vi "Photobleach Custom.vi"(8 "error in (no error)":errorcluster, 9 "Shutter Enable":bool[](array[boolean]), 10 "Length (mm)":dbl, 11 "Application in":refnum<class "Application.lvclass">) -> (0 "error out":errorcluster, 3 "Application out":refnum<class "Application.lvclass">)   [LabVIEW 2018, in "Application.lvlib" / "Application.lvclass"]
uses:
  Application.lvclass
  Application Messages/Close Shutter Msg/Close Shutter Msg.lvclass
  C:/Program Files/National Instruments/LabVIEW 2018/vi.lib/ActorFramework/Message/Message.lvclass
  Application.lvclass/Application.ctl
  Hardware/Laser Messages/Set Laser Power Msg/Set Laser Power Msg.lvclass/Set Laser Power Msg.ctl
  <vilib>/ActorFramework/Message Enqueuer/Message Enqueuer.lvclass/Message Enqueuer.ctl
  Hardware/Stage Controller Messages/Photobleach Custom Msg/Photobleach Custom Msg.lvclass/Photobleach Custom Msg.ctl
  <vilib>/ActorFramework/Message Enqueuer/Enqueue.vi
  Hardware/Laser Messages/Set Laser Power Msg/Set Laser Power Msg.lvclass
  Hardware/Stage Controller Messages/Photobleach Custom Msg/Photobleach Custom Msg.lvclass
  Resources/GLOBAL/GLOBAL Time-critical.vi
  <vilib>/ActorFramework/Message Priority Queue/Priority Enqueue.vi
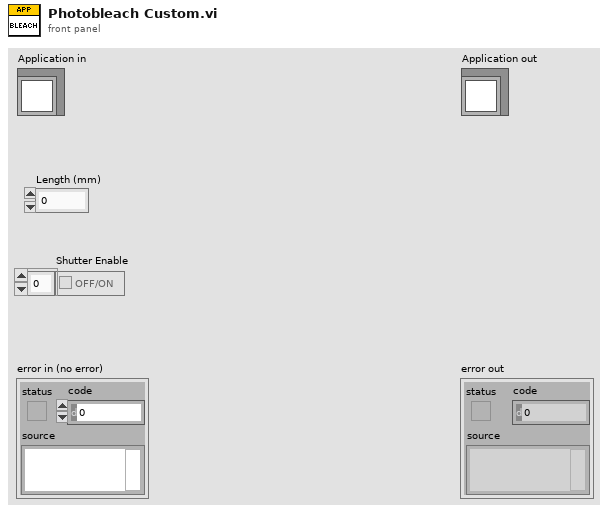
[diagram p1: front panel]
types:
  T1 = typedef "Shutter Configuration.ctl" = cluster{"IO Line":tag, "Name":string, "Wavelength":u16, "Max rate (Hz)":dbl}
  T2 = typedef "Laser Configuration.ctl" = cluster{"Serial Port":refnum<visa-resource-name>, "Laser Type":enum16{"Disable", "Laser Quantum", "Coherent OBIS", "PRM1-Z8", "Coherent HOPS"}, "Polarizer Amplitude":dbl, "Polarizer Theta Zero":dbl, "Wavelength":u16}
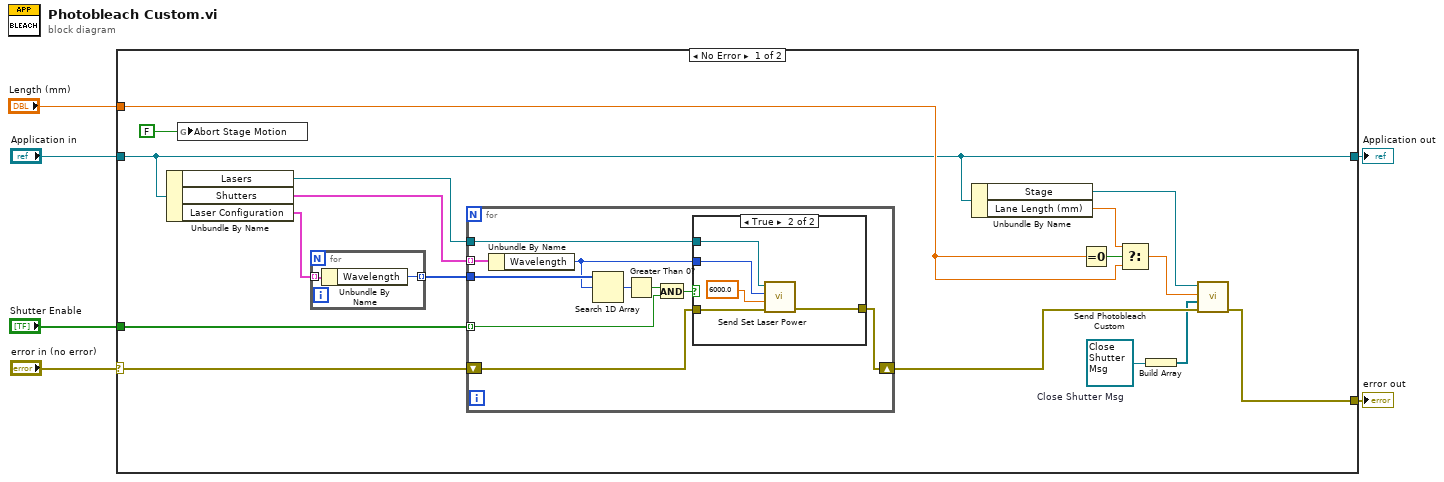
[diagram p0: block diagram]
diagram:
  n1 = case shown="No Error" "error in (no error)" {
    selector: "error in (no error)" -> [w16 w43]
    tunnel: [w22 w43] -> w5
    tunnel: [w14 w42] -> w3
    tunnel: "Application in" -> [w14 w42]
    tunnel: "Length (mm)" -> [w18 _]
    tunnel: "Shutter Enable" -> [w11 _]
    frame No Error {
      w7 = refnum<class "Close Shutter Msg.lvclass"> refnum  # Close Shutter Msg
      n2 = Unbundle By Name(w14) -> ("Lasers"=w13:refnum<class "Message Enqueuer.lvclass">, "Shutters"=w12:T1[], "Laser Configuration"=w10:T2[])
      n3 = global write "GLOBAL Time-critical.vi" "Abort Stage Motion"(FALSE ("Abort Stage Motion")) -> ()
      n4 = for {
        tunnel: w10 -> [w25] mode=indexing
        tunnel: [w24] -> w9 mode=indexing
        n5 = Unbundle By Name(w25) -> ("Wavelength"=w24:u16)
      }
      n6 = for {
        shift-right: [w34] -> w15
        shift-left: w16 -> [w35]
        tunnel: w13 -> [w33]
        tunnel: w12 -> [w32] mode=indexing
        tunnel: w11 -> [w28] mode=indexing
        tunnel: w9 -> [w31]
        n7 = Unbundle By Name(w32) -> ("Wavelength"=w30:u16)
        n8 = Search 1D Array(1D array=w31, element=w30) -> (index of element=w26:i32)  [unwired: 1 in]
        n9 = Greater Than 0?(x=w26) -> (x > 0?=w27:bool)
        n10 = And(x=w27, y=w28) -> (x .and. y?=w29:bool)
        n11 = case shown="True" w29 {
          tunnel: w35 -> [w36 w41]
          tunnel: [w36 w40] -> w34
          tunnel: w33 -> [_ w39]
          tunnel: w30 -> [_ w37]
          frame False {
          }
          frame True {
            n12 = call "Send Set Laser Power.vi"("error in (no error)"=w41, "Power"=6000.0, "Wavelength"=w37, "Message Enqueuer"=w39) -> ("error out"=w40:errorcluster)  [unwired: 6 in, 1 out]
          }
        }
      }
      n13 = Unbundle By Name(w14) -> ("Stage"=w23:refnum<class "Message Enqueuer.lvclass">, "Lane Length (mm)"=w20:dbl)
      n14 = Equal To 0?(x=w18) -> (x = 0?=w17:bool)
      n15 = Select(t=w20, s=w17, f=w18) -> (s? t:f=w19:dbl)
      n16 = Build Array(w7) -> (w8:refnum<class "Close Shutter Msg.lvclass">[])
      n17 = call "Send Photobleach Custom.vi"("error in (no error)"=w15, "Reply"=w8, "Custom Length"=w19, "Message Enqueuer"=w23) -> ("error out"=w22:errorcluster)  [unwired: 6 in, 1 out]
    }
    frame Error {
    }
  }
  "error out" <- w5
  "Application out" <- w3
